vi "Stop.vi"(8 "error in (no error)":errorcluster, 10 "Message in":refnum<class "StopMessage.lvclass">, 11 "Waveform in":refnum<class "Waveform.lvclass">) -> (0 "error out":errorcluster, 3 "Waveform out":refnum<class "Waveform.lvclass">)   [LabVIEW 2012, in "Waveform.lvclass"]
doc: "This member function is called when the statemachine in the run.vi receives an 'stop' command. It relays the message to all observers of the component.\n\nOverride this member function in your derived class if you need additional stop functionality (but don't forget to call the parent method)."
uses:
  Waveform.lvclass
  <vilib>/Distrio/Murmex/StopMessage/StopMessage.lvclass
  <vilib>/Distrio/Murmex/Murmex/Murmex.lvclass
  Waveform.lvclass/Waveform.ctl
panel:
  # "This method is called when the STOP\ntrigger is sent. \n\nOverride this method when your component needs to\nrespond to this trigger. \n\nCall parent for proper implementation"
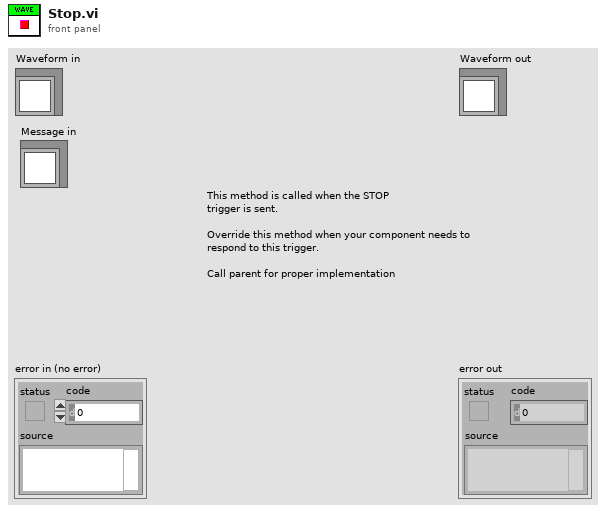
[diagram p1: front panel]
types:
  T1 = enum8{"Enabled", "Disabled", "Disabled and Grayed Out"}
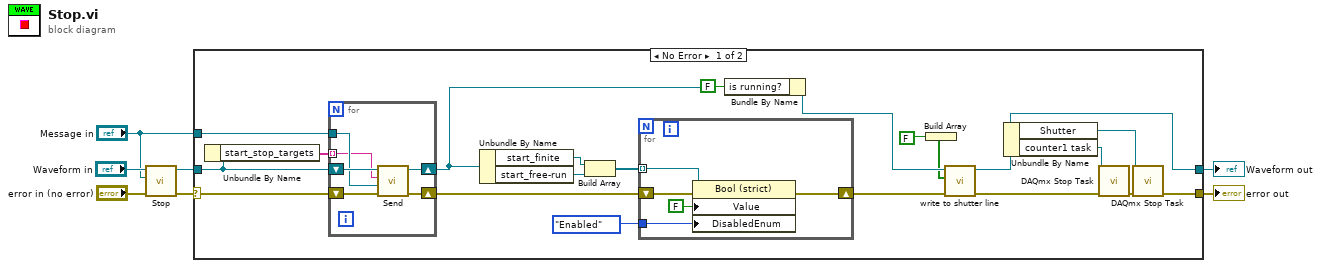
[diagram p0: block diagram]
diagram:
  n1 = call-parent "Stop.vi"("error in (no error)"="error in (no error)", "Message in"="Message in", "Murmex in"="Waveform in") -> ("error out"=w5:errorcluster, "Murmex out"=w4:refnum<class "Waveform.lvclass">)  [unwired: 7 in]
  n2 = case shown="No Error" w5 {
    selector: w5 -> [w23 w40]
    tunnel: w4 -> [w19 w41]
    tunnel: [w10 w41] -> w3
    tunnel: [w15 w40] -> w2
    tunnel: "Message in" -> [w20 _]
    frame No Error {
      n3 = Unbundle By Name(w19) -> ("start_stop_targets"=w18:string[])
      n4 = for {
        shift-right: [w31] -> w22
        shift-left: w23 -> [w32]
        shift-right: [w33] -> w21
        shift-left: w19 -> [w34]
        tunnel: w20 -> [w30]
        tunnel: w18 -> [w29] mode=indexing
        n5 = call <vilib>:"Send.vi"("error in (no error)"=w32, "Message"=w30, "recipient"=w29, "Murmex in"=w34) -> ("error out"=w31:errorcluster, "Murmex out"=w33:refnum<class "Waveform.lvclass">)  [unwired: 6 in]
      }
      n6 = Unbundle By Name(w21) -> ("start_finite"=w27:refnum<vi>, "start_free-run"=w28:refnum<vi>)
      n7 = Build Array(w27, w28) -> (w26:refnum<vi>[])
      n8 = for {
        tunnel: w26 -> [w38] mode=indexing
        shift-right: [w35] -> w13
        shift-left: w22 -> [w39]
        tunnel: T1."Enabled" ("Disabled") -> [w36]
        n9 = property class="Bool (strict)"(reference=w38, error in=w39, "Value"=FALSE, "DisabledEnum"=w36) -> (error out=w35:errorcluster)  [unwired: 1 out]
      }
      n10 = Bundle By Name(cluster=w21, "is running?"=FALSE ("runtime.is running?")) -> (w11:refnum<class "Waveform.lvclass">)
      n11 = Build Array(FALSE) -> (w8:bool[])
      n12 = call-dynamic "write to shutter line.vi"("error in (no error)"=w13, "Output Array"=w8, "Waveform in"=w11) -> ("error out"=w12:errorcluster, "Waveform out"=w10:refnum<class "Waveform.lvclass">)  [unwired: 7 in]
      n13 = Unbundle By Name(w10) -> ("Shutter"=w14:refnum<k21>, "counter1 task"=w17:refnum<k21>)
      n14 = call <vilib>:"DAQmx Stop Task.vi"("task/channels in"=w17, "error in"=w12) -> ("error out"=w16:errorcluster)  [unwired: 12 in, 1 out]
      n15 = call <vilib>:"DAQmx Stop Task.vi"("task/channels in"=w14, "error in"=w16) -> ("error out"=w15:errorcluster)  [unwired: 12 in, 1 out]
    }
    frame Error {
    }
  }
  "error out" <- w2
  "Waveform out" <- w3
